vi "Example.vi"() -> ()   [LabVIEW 2015, in "SLSC Switch.lvlib"]
uses:
  SLSC Switch.lvlib
  Classes/SLSC Switch/SLSC Switch.lvclass
  Classes/slscsl/RelayAction.ctl
  Classes/slscsl/slscsl.lvclass
  Classes/slscsl/RelayPosition.ctl
  Classes/SLSC Switch/Disconnect Channels (Multiple).vi
  Classes/SLSC Switch/Connect Channels (Single).vi
  Classes/SLSC Switch/Connect Channels (Multiple).vi
  Classes/SLSC Switch/Disconnect Channels (Single).vi
  <vilib>/SLSC/SLSC.lvlib
  <vilib>/SLSC/Flatten Names (String).vi
  Classes/SLSC Switch/Initialize (Remote).vi
panel:
  in  "https?":bool
  in  "Port":u16=8001
  in  "Hostname/IP":string="localhost"
  in  "suffix":string
  in  "Add Topology":bool
  in  "Disconnect All":bool
  out "Active Connections":i32(listbox)
  in  "Tab Control":T1(tab)
  in  "Available Relays":i32[](listbox)
  in  "Open":bool
  in  "Close":bool
  in  "Channel A":i32(listbox)=-1
  in  "Channel B":i32(listbox)=-1
  in  "Disconnect":bool
  in  "Connect":bool
  in  "Add to List":bool
  in  "Connection List":string
  in  "Disconnect Multiple":bool
  in  "Connect Multiple":bool
  in  "Channel B":i32(listbox)=-1
  in  "Channel A":i32(listbox)=-1
  in  "Check MUXList":bool
  in  "Add to MUXList":bool
  in  "Remove from MUXList":bool
  in  "Destinations":i32[](listbox)
  in  "Source":i32(listbox)=-1
  out "Relay Status":cluster{"RelayPosition":T2, "Name":string}[](array[cluster]) {"RelayPosition" items=["Open"=10, "Closed"=11]}
  out "error out":errorcluster
  in  "stop":bool
  in  "error in (no error)":errorcluster
  in  "Topology":string
  in  "device":refnum<k21>
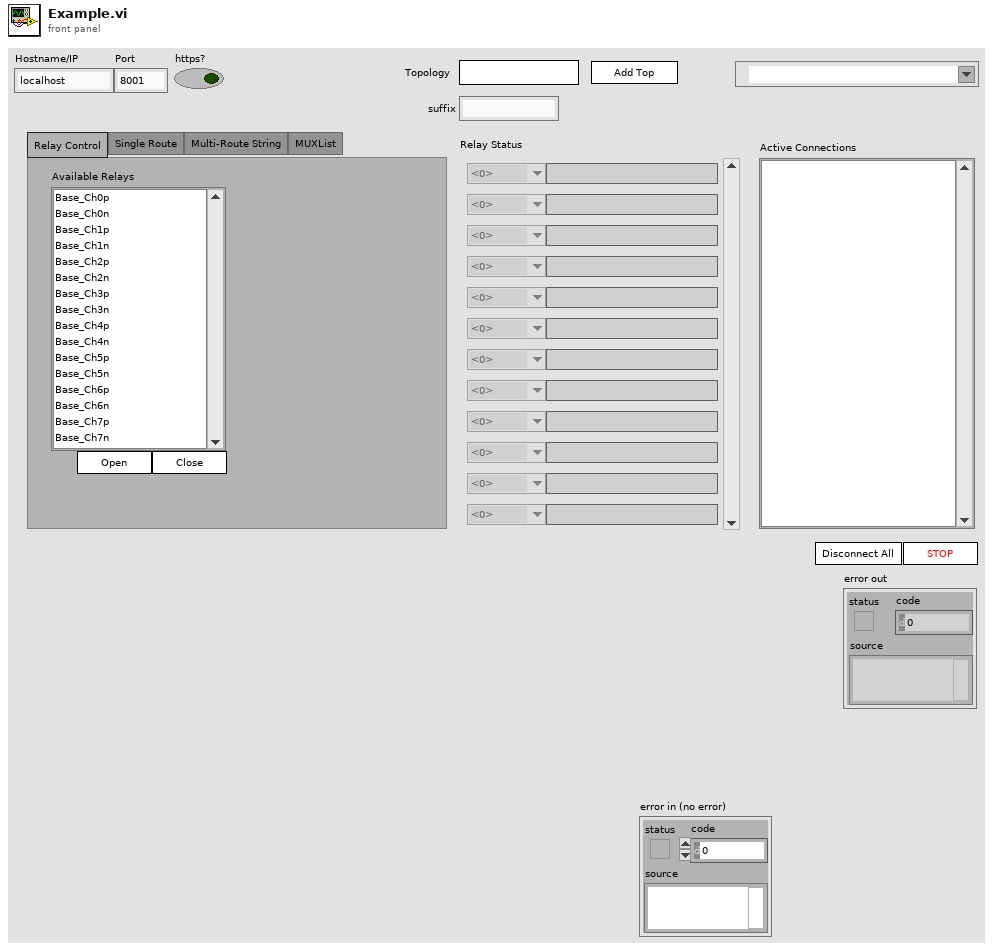
[diagram p1: front panel]
types:
  T1 = enum32{"Relay Control", "Single Route", "Multi-Route String", "MUXList"}
  T2 = typedef "SLSC Switch.lvlib/slscsl.lvclass/RelayPosition.ctl" = i32
  T3 = typedef "SLSC Switch.lvlib/SLSC Switch.lvclass/Connection.ctl" = cluster{"channel 1":string, "channel 2":string}
  T4 = typedef "SLSC Switch.lvlib/slscsl.lvclass/RelayAction.ctl" = u32
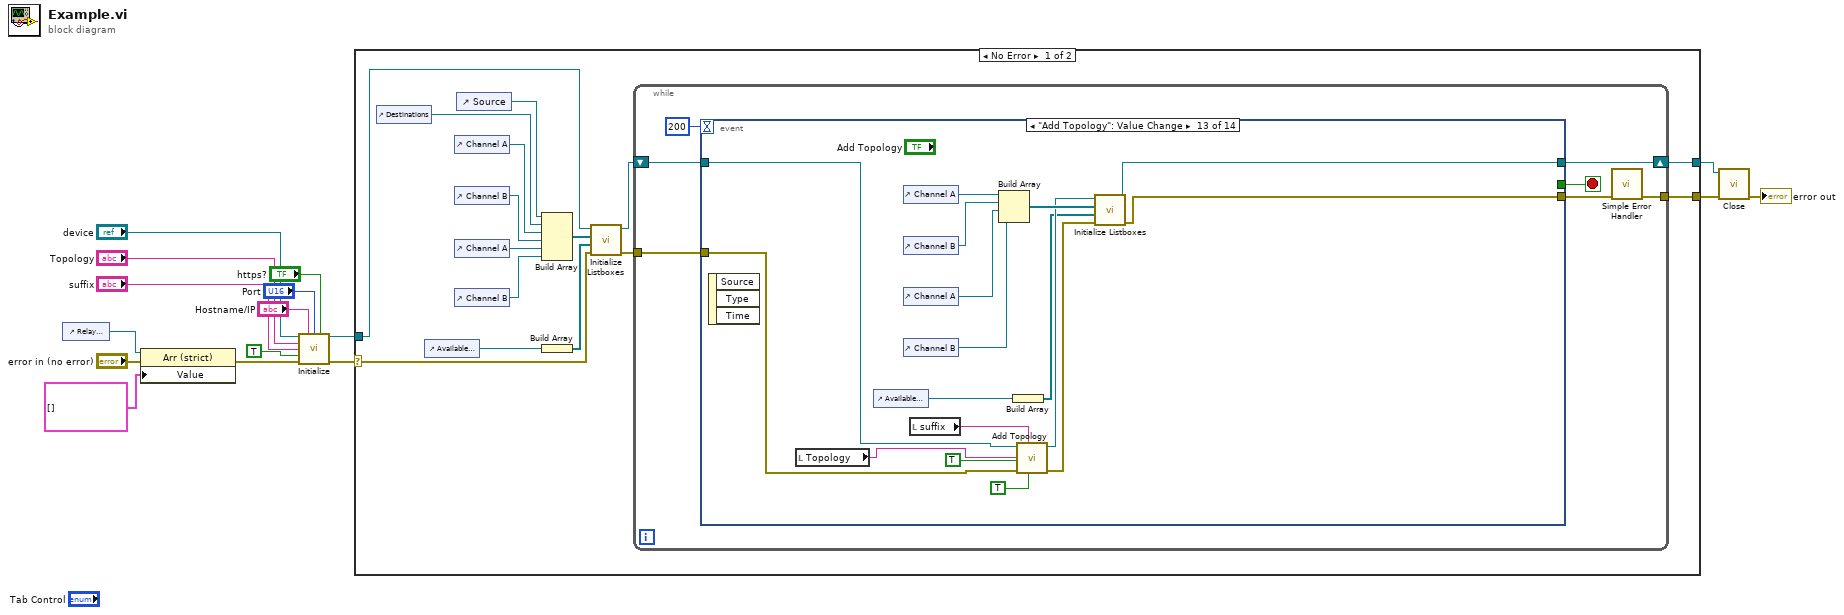
[diagram p0: block diagram]
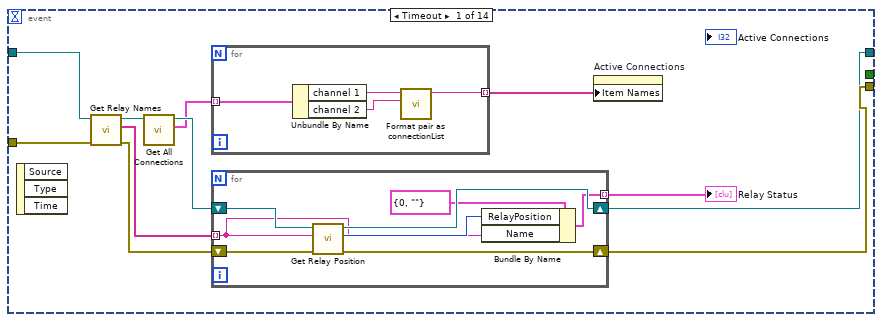
[diagram p2: hidden frame]
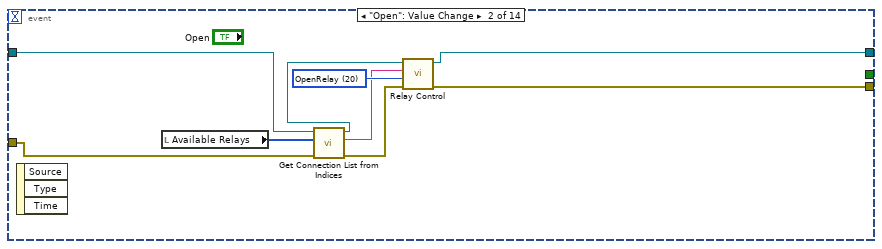
[diagram p3: hidden frame]
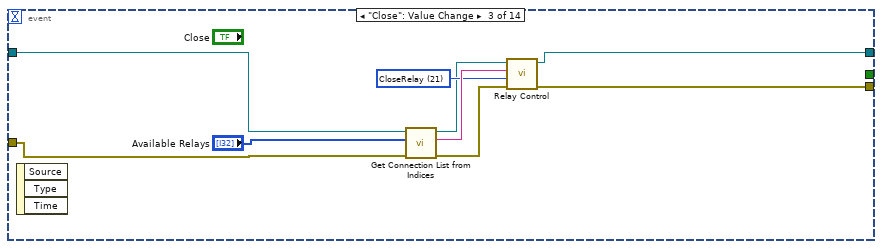
[diagram p4: hidden frame]
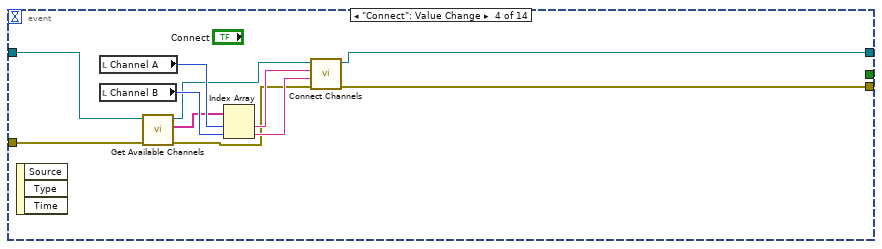
[diagram p5: hidden frame]
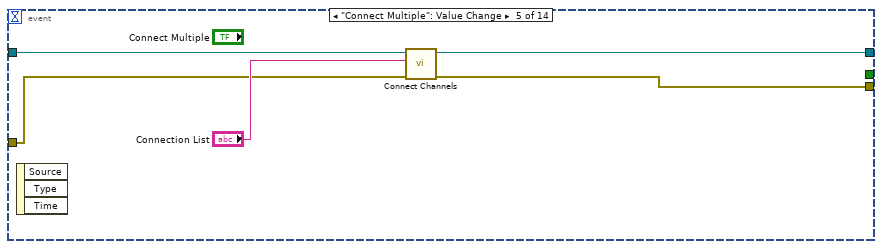
[diagram p6: hidden frame]
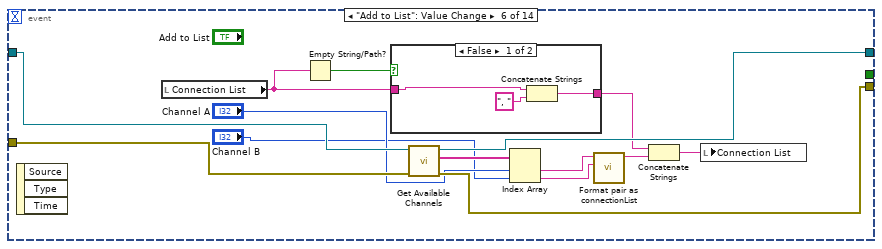
[diagram p7: hidden frame]
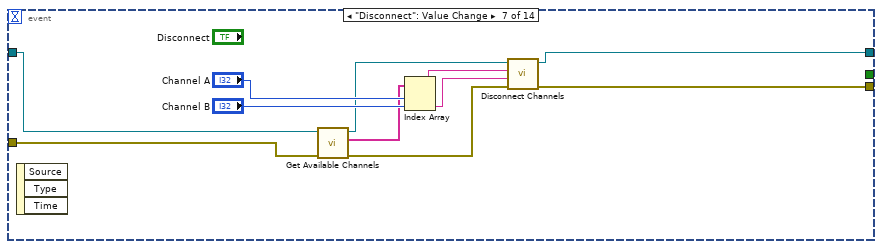
[diagram p9: hidden frame]
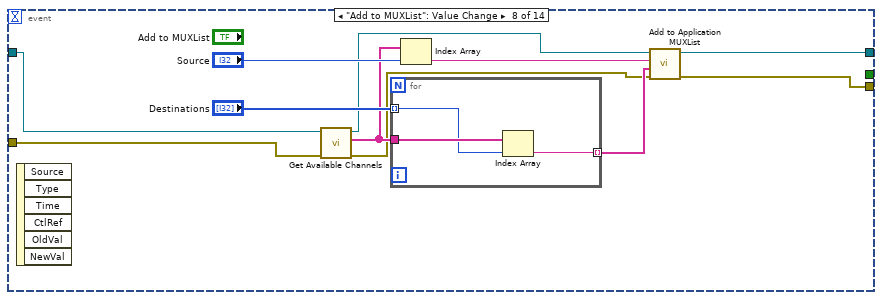
[diagram p10: hidden frame]
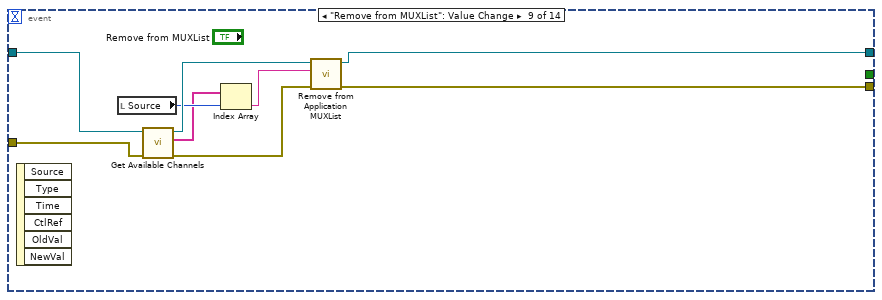
[diagram p11: hidden frame]
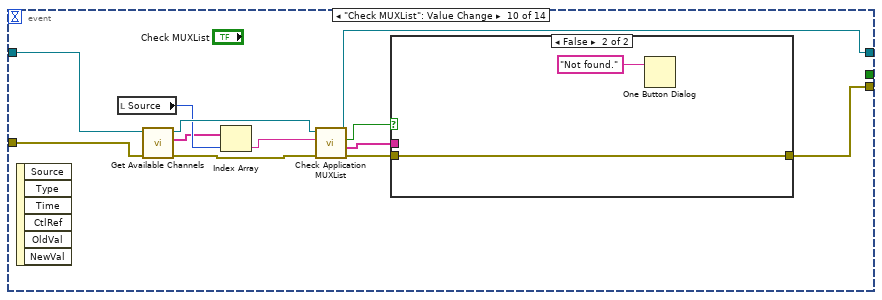
[diagram p12: hidden frame]
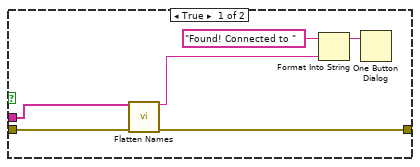
[diagram p13: hidden frame]
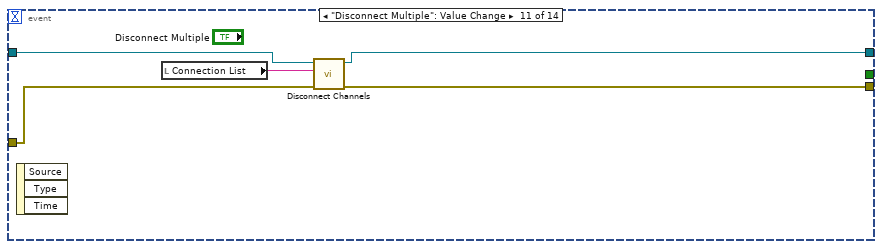
[diagram p14: hidden frame]
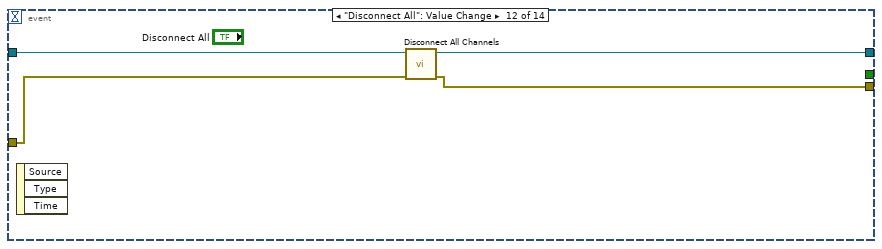
[diagram p15: hidden frame]
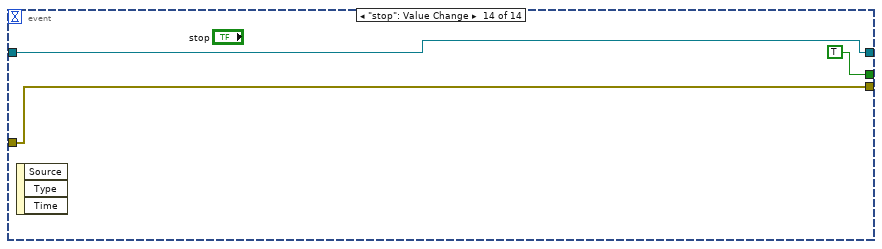
[diagram p16: hidden frame]
diagram:
  n1 = control-ref of="Relay Status"() -> (w8:refnum<vi>)
  n2 = property class="Arr (strict)"(reference=w8, error in="error in (no error)", "Value"=cluster{"RelayPosition":T2, "Name":string}[] []) -> (error out=w6:errorcluster)  [unwired: 1 out]
  n3 = call-poly "Initialize.vi"("device"="device", "Hostname/IP"="Hostname/IP", "Port"="Port", "https?"="https?", "Topology"="Topology", "topology suffix (none)"="suffix", "reset device (boolean value)"=TRUE, "error in (no error)"=w6) -> ("SLSC Switch out"=w11:refnum<class "SLSC Switch.lvclass">, "error out"=w12:errorcluster)  [unwired: 6 in]
  n4 = case shown="No Error" w12 {
    selector: w12 -> [w21 w197]
    tunnel: [w31 w197] -> w15
    tunnel: [w30 w198] -> w14
    tunnel: w11 -> [w28 w198]
    frame No Error {
      n5 = control-ref of="Destinations"() -> (w17:refnum<vi>)
      n6 = control-ref of="Available Relays"() -> (w22:refnum<vi>)
      n7 = control-ref of="Channel A"() -> (w26:refnum<vi>)
      n8 = control-ref of="Channel B"() -> (w25:refnum<vi>)
      n9 = control-ref of="Channel A"() -> (w24:refnum<vi>)
      n10 = control-ref of="Channel B"() -> (w23:refnum<vi>)
      n11 = control-ref of="Source"() -> (w18:refnum<vi>)
      n12 = Build Array(w18, w17, w26, w25, w24, w23) -> (w20:refnum<vi>[])
      n13 = Build Array(w22) -> (w19:refnum<vi>[])
      n14 = call "Initialize Listboxes.vi"("error in (no error)"=w21, "Relay Boxes"=w19, "Channel Boxes"=w20, "SLSC Switch in"=w28) -> ("error out"=w27:errorcluster, "SLSC Switch out"=w29:refnum<class "SLSC Switch.lvclass">)  [unwired: 6 in]
      n15 = while {
        shift-right: [w36] -> w30
        shift-left: w29 -> [w37]
        tunnel: w27 -> [w38]
        tunnel: [w32] -> w31
        stop <- w34 stop-if-true
        n16 = event shown="[12] \"Add Topology\": Value Change" {
          selector: _ -> [_ _ _ _ _ _ _ _ _ _ _ _ _ _]
          dyn-events: _ -> [_ _ _ _ _ _ _ _ _ _ _ _ _ _]
          timeout: 200 -> [_ _ _ _ _ _ _ _ _ _ _ _ _ _]
          tunnel: w38 -> [w40 w63 w72 w81 w92 w108 w115 w126 w140 w153 w170 w176 w192 w196]
          tunnel: [w49 w70 w79 w89 w91 w106 w123 w127 w143 w148 w169 w173 w180 w196] -> w33
          tunnel: w37 -> [w43 w67 w74 w84 w95 w109 w118 w135 w147 w159 w172 w175 w193 w195]
          tunnel: [w48 w69 w78 w90 w94 w107 w124 w130 w145 w157 w171 w174 w182 w195] -> w36
          tunnel: [_ _ _ _ _ _ _ _ _ _ _ _ _ TRUE] -> w34
          event Timeout {
            n17 = event-data() -> ()  [unwired: 1 in, 3 out]
            n18 = call "Get Relay Names.vi"("error in (no error)"=w40, "SLSC Switch in"=w43) -> ("error out"=w39:errorcluster, "Relay Names"=w41:string[], "SLSC Switch out"=w42:refnum<class "SLSC Switch.lvclass">)  [unwired: 7 in]
            n19 = call "Get All Connections.vi"("Route Manager in"=w42) -> ("connections"=w45:T3[], "Route Manager out"=w47:refnum<class "SLSC Switch.lvclass">)  [unwired: 9 in]
            n20 = for {
              tunnel: w45 -> [w53] mode=indexing
              tunnel: [w50] -> w44 mode=indexing
              n21 = Unbundle By Name(w53) -> ("channel 1"=w52:string, "channel 2"=w51:string)
              n22 = call "Format pair as connectionList.vi"("channel in"=w51, "channel 1"=w52) -> ("connectionList"=w50:string)  [unwired: 9 in]
            }
            n23 = for {
              shift-right: [w58] -> w48
              shift-left: w47 -> [w61]
              shift-right: [w59] -> w49
              shift-left: w39 -> [w60]
              tunnel: [w55] -> w46 mode=indexing
              tunnel: w41 -> [w54] mode=indexing
              n24 = call "Get Relay Position.vi"("error in (no error)"=w60, "relay name"=w54, "SLSC Switch in"=w61) -> ("error out"=w59:errorcluster, "position"=w56:T2, "SLSC Switch out"=w58:refnum<class "SLSC Switch.lvclass">)  [unwired: 6 in]
              n25 = Bundle By Name(cluster=cluster{"RelayPosition":T2, "Name":string} {"RelayPosition"=0, "Name"=""} ("Relay"), "RelayPosition"=w56, "Name"=w54) -> (w55:cluster{"RelayPosition":T2, "Name":string})
            }
            "Relay Status" <- w46
            n26 = property on="Active Connections" class="LstBox (strict)"("Item Names"=w44) -> ()  [unwired: 2 in, 2 out]
          }
          event "Open": Value Change {
            w68 = T4 20 items=["CloseRelay"=21, "OpenRelay"=20] ("RelayAction")
            n27 = event-data() -> ()  [unwired: 1 in, 3 out]
            n28 = local read "Available Relays"() -> (w64:i32[])
            n29 = call "Get Connection List from Indices.vi"("error in (no error)"=w63, "Available Relays"=w64, "SLSC Switch in"=w67) -> ("error out"=w62:errorcluster, "String"=w65:string, "SLSC Switch out"=w66:refnum<class "SLSC Switch.lvclass">)  [unwired: 6 in]
            n30 = call "Relay Control.vi"("error in (no error)"=w62, "relay action"=w68, "relay names"=w65, "SLSC Switch in"=w66) -> ("error out"=w70:errorcluster, "SLSC Switch out"=w69:refnum<class "SLSC Switch.lvclass">)  [unwired: 6 in]
          }
          event "Close": Value Change {
            w76 = T4 21 items=["CloseRelay"=21, "OpenRelay"=20] ("RelayAction")
            n31 = event-data() -> ()  [unwired: 1 in, 3 out]
            n32 = call "Get Connection List from Indices.vi"("error in (no error)"=w72, "Available Relays"="Available Relays", "SLSC Switch in"=w74) -> ("error out"=w71:errorcluster, "String"=w77:string, "SLSC Switch out"=w73:refnum<class "SLSC Switch.lvclass">)  [unwired: 6 in]
            n33 = call "Relay Control.vi"("error in (no error)"=w71, "relay action"=w76, "relay names"=w77, "SLSC Switch in"=w73) -> ("error out"=w79:errorcluster, "SLSC Switch out"=w78:refnum<class "SLSC Switch.lvclass">)  [unwired: 6 in]
          }
          event "Connect": Value Change {
            n34 = event-data() -> ()  [unwired: 1 in, 3 out]
            n35 = local read "Channel A"() -> (w86:i32)
            n36 = local read "Channel B"() -> (w85:i32)
            n37 = call "Get Available Channels.vi"("error in (no error)"=w81, "SLSC Switch in"=w84) -> ("error out"=w80:errorcluster, "Channels"=w82:string[], "SLSC Switch out"=w83:refnum<class "SLSC Switch.lvclass">)  [unwired: 7 in]
            n38 = Index Array(array=w82, index #1=w86, index #2=w85) -> (element #1=w88:string, element #2=w87:string)
            n39 = call-poly "Connect Channels.vi"("error in (no error)"=w80, "channel 2"=w87, "channel 1"=w88, "SLSC Switch in"=w83) -> ("error out"=w89:errorcluster, "SLSC Switch out"=w90:refnum<class "SLSC Switch.lvclass">)  [unwired: 6 in]
          }
          event "Connect Multiple": Value Change {
            n40 = event-data() -> ()  [unwired: 1 in, 3 out]
            n41 = call-poly "Connect Channels.vi"("error in (no error)"=w92, "connection list"="Connection List", "SLSC Switch in"=w95) -> ("error out"=w91:errorcluster, "SLSC Switch out"=w94:refnum<class "SLSC Switch.lvclass">)  [unwired: 7 in]
          }
          event "Add to List": Value Change {
            n42 = event-data() -> ()  [unwired: 1 in, 3 out]
            n43 = local read "Connection List"() -> (w103:string)
            n44 = Empty String/Path?(string/path=w103) -> (empty?=w104:bool)
            n45 = case shown="False" w104 {
              tunnel: w103 -> [w112 w113]
              tunnel: [w110 w113] -> w102
              frame False {
                n46 = Concatenate Strings(w112, ", " ("string")) -> (w110:string)
              }
              frame True {
              }
            }
            n47 = call "Get Available Channels.vi"("error in (no error)"=w108, "SLSC Switch in"=w109) -> ("error out"=w106:errorcluster, "Channels"=w105:string[], "SLSC Switch out"=w107:refnum<class "SLSC Switch.lvclass">)  [unwired: 7 in]
            n48 = Index Array(array=w105, index #1="Channel A", index #2="Channel B") -> (element #1=w101:string, element #2=w100:string)
            n49 = call "Format pair as connectionList.vi"("channel in"=w100, "channel 1"=w101) -> ("connectionList"=w99:string)  [unwired: 9 in]
            n50 = Concatenate Strings(w102, w99) -> (w98:string)
            n51 = local write "Connection List"(w98) -> ()
          }
          event "Disconnect": Value Change {
            n52 = event-data() -> ()  [unwired: 1 in, 3 out]
            n53 = call "Get Available Channels.vi"("error in (no error)"=w115, "SLSC Switch in"=w118) -> ("error out"=w114:errorcluster, "Channels"=w117:string[], "SLSC Switch out"=w116:refnum<class "SLSC Switch.lvclass">)  [unwired: 7 in]
            n54 = Index Array(array=w117, index #1="Channel A", index #2="Channel B") -> (element #1=w122:string, element #2=w121:string)
            n55 = call-poly "Disconnect Channels.vi"("error in (no error)"=w114, "channel 2"=w121, "channel 1"=w122, "SLSC Switch in"=w116) -> ("error out"=w123:errorcluster, "SLSC Switch out"=w124:refnum<class "SLSC Switch.lvclass">)  [unwired: 6 in]
          }
          event "Add to MUXList": Value Change {
            n56 = event-data() -> ()  [unwired: 1 in, 6 out]
            n57 = call "Get Available Channels.vi"("error in (no error)"=w126, "SLSC Switch in"=w135) -> ("error out"=w125:errorcluster, "Channels"=w132:string[], "SLSC Switch out"=w131:refnum<class "SLSC Switch.lvclass">)  [unwired: 7 in]
            n58 = for {
              tunnel: "Destinations" -> [w136] mode=indexing
              tunnel: w132 -> [w138]
              tunnel: [w137] -> w128 mode=indexing
              n59 = Index Array(array=w138, index=w136) -> (element=w137:string)
            }
            n60 = Index Array(array=w132, index="Source") -> (element=w129:string)
            n61 = call "Add to Application MUXList.vi"("error in (no error)"=w125, "Destinations"=w128, "Source"=w129, "SLSC Switch in"=w131) -> ("error out"=w127:errorcluster, "SLSC Switch out"=w130:refnum<class "SLSC Switch.lvclass">)  [unwired: 5 in, 1 out]
          }
          event "Remove from MUXList": Value Change {
            n62 = event-data() -> ()  [unwired: 1 in, 6 out]
            n63 = local read "Source"() -> (w142:i32)
            n64 = call "Get Available Channels.vi"("error in (no error)"=w140, "SLSC Switch in"=w147) -> ("error out"=w139:errorcluster, "Channels"=w141:string[], "SLSC Switch out"=w146:refnum<class "SLSC Switch.lvclass">)  [unwired: 7 in]
            n65 = Index Array(array=w141, index=w142) -> (element=w144:string)
            n66 = call "Remove from Application MUXList.vi"("error in (no error)"=w139, "Source"=w144, "SLSC Switch in"=w146) -> ("error out"=w143:errorcluster, "SLSC Switch out"=w145:refnum<class "SLSC Switch.lvclass">)  [unwired: 7 in]
          }
          event "Check MUXList": Value Change {
            n67 = event-data() -> ()  [unwired: 1 in, 6 out]
            n68 = local read "Source"() -> (w155:i32)
            n69 = call "Get Available Channels.vi"("error in (no error)"=w153, "SLSC Switch in"=w159) -> ("error out"=w152:errorcluster, "Channels"=w154:string[], "SLSC Switch out"=w158:refnum<class "SLSC Switch.lvclass">)  [unwired: 7 in]
            n70 = Index Array(array=w154, index=w155) -> (element=w156:string)
            n71 = call "Check Application MUXList.vi"("error in (no error)"=w152, "Source"=w156, "SLSC Switch in"=w158) -> ("error out"=w149:errorcluster, "Destinations"=w151:string[], "found?"=w150:bool, "SLSC Switch out"=w157:refnum<class "SLSC Switch.lvclass">)  [unwired: 4 in, 1 out]
            n72 = case shown="False" w150 {
              tunnel: w151 -> [w163 _]
              tunnel: w149 -> [w161 w166]
              tunnel: [w160 w166] -> w148
              frame True {
                n73 = call-poly <vilib>:"Flatten Names.vi"("names in"=w163, "error in (no error)"=w161) -> ("names out"=w162:string, "error out"=w160:errorcluster)  [unwired: 12 in]
                n74 = Format Into String(initial string="Found! Connected to ", w162) -> (resulting string=w164:string)  [unwired: 2 in, 1 out]
                n75 = One Button Dialog(message=w164) -> ()  [unwired: 1 in, 1 out]
              }
              frame False {
                n76 = One Button Dialog(message="Not found.") -> ()  [unwired: 1 in, 1 out]
              }
            }
          }
          event "Disconnect Multiple": Value Change {
            n77 = event-data() -> ()  [unwired: 1 in, 3 out]
            n78 = local read "Connection List"() -> (w168:string)
            n79 = call-poly "Disconnect Channels.vi"("error in (no error)"=w170, "disconnection list"=w168, "SLSC Switch in"=w172) -> ("error out"=w169:errorcluster, "SLSC Switch out"=w171:refnum<class "SLSC Switch.lvclass">)  [unwired: 7 in]
          }
          event "Disconnect All": Value Change {
            n80 = event-data() -> ()  [unwired: 1 in, 3 out]
            n81 = call "Disconnect All Channels.vi"("error in (no error)"=w176, "SLSC Switch in"=w175) -> ("error out"=w173:errorcluster, "SLSC Switch out"=w174:refnum<class "SLSC Switch.lvclass">)  [unwired: 8 in]
          }
          event "Add Topology": Value Change {
            n82 = event-data() -> ()  [unwired: 1 in, 3 out]
            n83 = local read "Topology"() -> (w190:string)
            n84 = control-ref of="Available Relays"() -> (w188:refnum<vi>)
            n85 = control-ref of="Channel A"() -> (w184:refnum<vi>)
            n86 = control-ref of="Channel B"() -> (w185:refnum<vi>)
            n87 = control-ref of="Channel A"() -> (w186:refnum<vi>)
            n88 = control-ref of="Channel B"() -> (w187:refnum<vi>)
            n89 = local read "suffix"() -> (w177:string)
            n90 = Build Array(w184, w185, w186, w187) -> (w189:refnum<vi>[])
            n91 = Build Array(w188) -> (w179:refnum<vi>[])
            n92 = call "Add Topology.vi"("Append to Active?"=TRUE, "topology suffix (none)"=w177, "error in (no error)"=w192, "reset device (boolean value)"=TRUE, "Topology"=w190, "SLSC Switch in"=w193) -> ("error out"=w181:errorcluster, "SLSC Switch out"=w183:refnum<class "SLSC Switch.lvclass">)  [unwired: 4 in]
            n93 = call "Initialize Listboxes.vi"("error in (no error)"=w181, "Relay Boxes"=w179, "Channel Boxes"=w189, "SLSC Switch in"=w183) -> ("error out"=w180:errorcluster, "SLSC Switch out"=w182:refnum<class "SLSC Switch.lvclass">)  [unwired: 6 in]
          }
          event "stop": Value Change {
            n94 = event-data() -> ()  [unwired: 1 in, 3 out]
          }
        }
        n95 = call <vilib>:"Simple Error Handler.vi"("error in (no error)"=w33) -> ("error out"=w32:errorcluster)  [unwired: 4 in, 4 out]
      }
    }
    frame Error {
    }
  }
  n96 = call "Close.vi"("error in (no error)"=w15, "SLSC Switch in"=w14) -> ("error out"=→"error out":errorcluster)  [unwired: 9 in]
